vi "EventClient_Create.vi"(8 "error in (no error)":errorcluster, 11 "Instance Name":string) -> (0 "error out":errorcluster, 3 "reference":T1)   [LabVIEW 2018]
uses:
  EventClient_ObjectReference.ctl
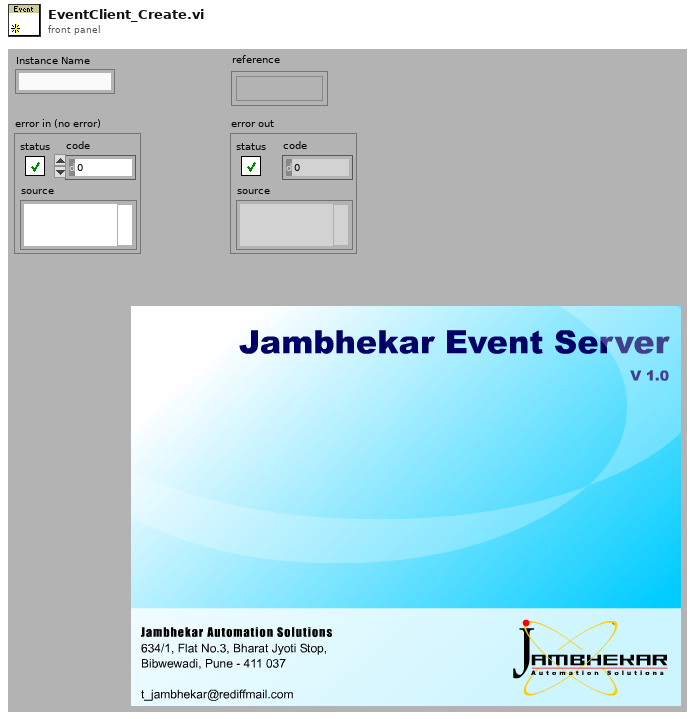
[diagram p1: front panel]
types:
  T1 = typedef "EventClient_ObjectReference.ctl" = refnum<k1>
  T2 = cluster{"Client":refnum<queue>, "Sub Events":string[], "PrvData":variant, "MyName":string}
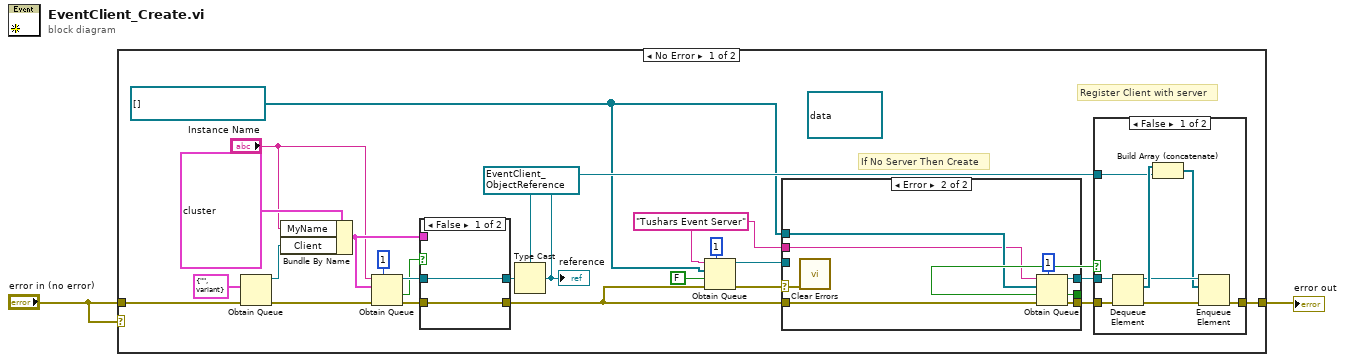
[diagram p0: block diagram]
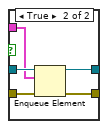
[diagram p2: hidden frame]
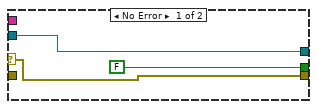
[diagram p3: hidden frame]
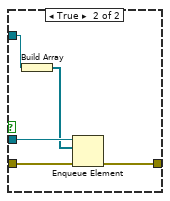
[diagram p4: hidden frame]
diagram:
  n1 = case shown="No Error" "error in (no error)" {
    tunnel: [w14 w59] -> w2
    tunnel: "error in (no error)" -> [w27 w59]
    frame No Error {
      w10 = T1[] [] items=["EventClient"]
      (unwired) refnum<queue> refnum ("queue out")
      w24 = T1 refnum items=["EventClient"] ("reference (default)")
      w5 = "Tushars Event Server" ("name (unnamed)")
      # "Register Client with server"
      # "If No Server Then Create"
      n2 = Obtain Queue(element data type=cluster{"Name":string, "Data":variant} {"Name"="", "Data"=variant} ("Cluster"), error in (no error)=w27) -> (queue out=w19:refnum<queue>, error out=w17:errorcluster)  [unwired: 2 in, 2 out]
      n3 = Bundle By Name(cluster=T2 {"Client"=refnum, "Sub Events"=[], "PrvData"=variant, "MyName"=""} ("data"), "MyName"="Instance Name", "Client"=w19) -> (w18:T2)
      n4 = Obtain Queue(max queue size (-1, unlimited)=1, name (unnamed)="Instance Name", element data type=w18, error in (no error)=w17) -> (queue out=w21:refnum<queue>, created new?=w3:bool, error out=w22:errorcluster)  [unwired: 1 in]
      n5 = case shown="False" w3 {
        tunnel: [w29 w34] -> w25
        tunnel: w22 -> [w28 w33]
        tunnel: w21 -> [w29 w32]
        tunnel: w18 -> [_ w31]
        tunnel: [w28 w30] -> w7
        frame False {
        }
        frame True {
          n6 = Enqueue Element(queue=w32, element=w31, error in (no error)=w33) -> (queue out=w34:refnum<queue>, error out=w30:errorcluster)  [unwired: 2 out]
        }
      }
      n7 = Type Cast(type=w24, x=w25) -> (*(type *) &x=w12:T1)
      "reference" <- w12
      n8 = Obtain Queue(max queue size (-1, unlimited)=1, name (unnamed)=w5, element data type=w10, create if not found? (T)=FALSE, error in (no error)=w7) -> (queue out=w6:refnum<queue>, error out=w8:errorcluster)  [unwired: 1 out]
      n9 = case shown="Error" w8 {
        selector: w8 -> [w35 w39]
        tunnel: [FALSE ("created new?") w45] -> w16
        tunnel: [w35 w44] -> w15
        tunnel: [w37 w43] -> w13
        tunnel: w10 -> [_ w41]
        tunnel: w7 -> [_ w38]
        tunnel: w6 -> [w37 _]
        tunnel: w5 -> [_ w40]
        frame No Error {
        }
        frame Error {
          n10 = call <vilib>:"Clear Errors.vi"("error in (no error)"=w39) -> ()  [unwired: 1 in, 6 out]
          n11 = Obtain Queue(max queue size (-1, unlimited)=1, name (unnamed)=w40, element data type=w41, error in (no error)=w38) -> (queue out=w43:refnum<queue>, created new?=w45:bool, error out=w44:errorcluster)  [unwired: 1 in]
        }
      }
      n12 = case shown="False" w16 {
        tunnel: w15 -> [w53 w58]
        tunnel: [w46 w57] -> w14
        tunnel: w13 -> [w52 w56]
        tunnel: w12 -> [w50 w55]
        frame False {
          n13 = Dequeue Element(queue=w52, error in (no error)=w53) -> (queue out=w49:refnum<queue>, element=w51:T1[], error out=w48:errorcluster)  [unwired: 2 out]
          n14 = Build Array (concatenate)(w51, w50) -> (w47:T1[])
          n15 = Enqueue Element(queue=w49, element=w47, error in (no error)=w48) -> (error out=w46:errorcluster)  [unwired: 3 out]
        }
        frame True {
          n16 = Build Array(w55) -> (w54:T1[])
          n17 = Enqueue Element(queue=w56, element=w54, error in (no error)=w58) -> (error out=w57:errorcluster)  [unwired: 3 out]
        }
      }
    }
    frame Error {
    }
  }
  "error out" <- w2
